vi "Extract subclasses from AUX device.vi"(9 "Data In":string, 10 "Class":string, 11 "Aux Device Settings in":T1 {"Signals"."% Open" min=0.0 max=100.0 step=0.1 format="%.4f"; "Signals"."Position" max=20.0 step=1.0 format="%.4f"; "Speed" max=7 step=1; "Gear" max=7 step=1; "Temp V Err" min=0.0 max=20.0 step=0.1; "Temp Err" min=0.0 max=20.0 step=0.1; "Scaling Factor" min=0.0 max=99.0 step=0.1; "Min Flow" min=0.0 max=20.0 step=0.1}) -> (1 "Data out":string, 3 "Aux Device Settings out":T1 {"Signals"."% Open" min=0.0 max=100.0 step=0.1 format="%.4f"; "Signals"."Position" max=20.0 step=1.0 format="%.4f"; "Speed" max=7 step=1; "Gear" max=7 step=1; "Temp V Err" min=0.0 max=20.0 step=0.1; "Temp Err" min=0.0 max=20.0 step=0.1; "Scaling Factor" min=0.0 max=99.0 step=0.1; "Min Flow" min=0.0 max=20.0 step=0.1})   [LabVIEW 2015, in "Mercury iXX.lvlib" / "Auxiliary.lvlib"]
uses:
  Auxiliary.lvlib
  Controls/AUX Device (Read).ctl
  Controls/Manufacturing Data.ctl
  Controls/AUX Signals (Read).ctl
  Mercury iXX.lvlib
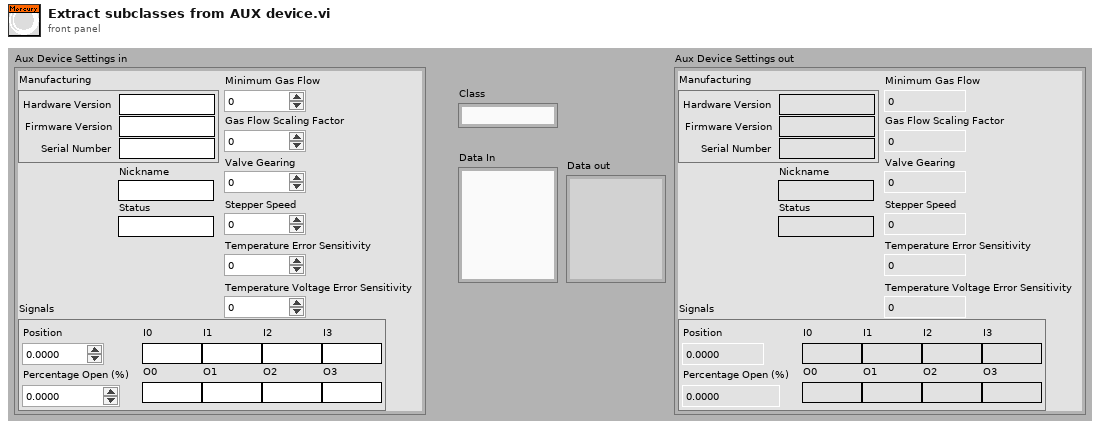
[diagram p1: front panel]
types:
  T1 = typedef "Mercury iXX.lvlib/Auxiliary.lvlib/AUX Device (Read).ctl" = cluster{"Manufacturing":T2, "Min Flow":dbl, "Scaling Factor":dbl, "Temp Err":dbl, "Temp V Err":dbl, "Gear":u32, "Speed":u32, "Signals":T3, "Nickname":string, "Status":string}
  T2 = typedef "Mercury iXX.lvlib/Manufacturing Data.ctl" = cluster{"Hardware Version":string, "Firmware Version":string, "Serial Number":string}
  T3 = typedef "Mercury iXX.lvlib/Auxiliary.lvlib/AUX Signals (Read).ctl" = cluster{"Position":dbl, "% Open":dbl, "I0":string, "I1":string, "I2":string, "I3":string, "O0":string, "O1":string, "O2":string, "O3":string}
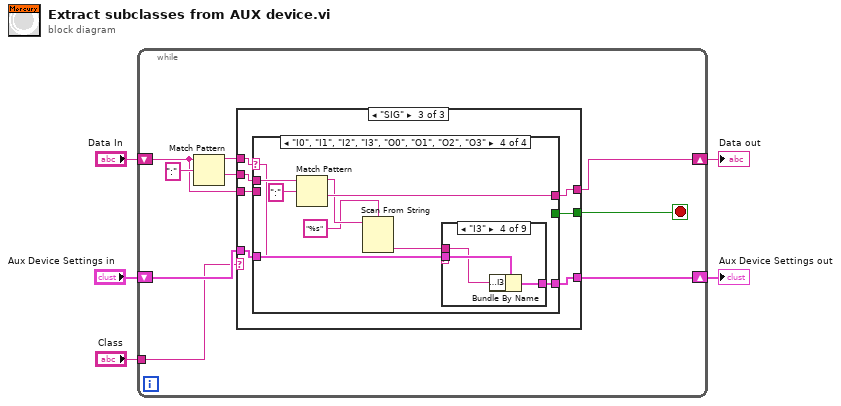
[diagram p0: block diagram]
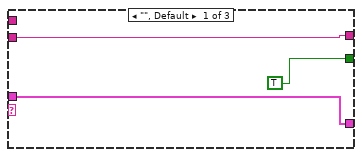
[diagram p2: hidden frame]
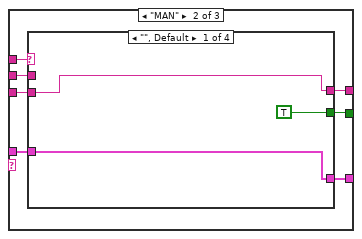
[diagram p3: hidden frame]
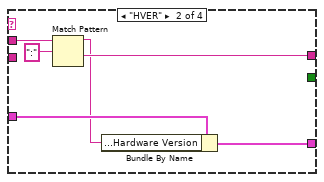
[diagram p4: hidden frame]
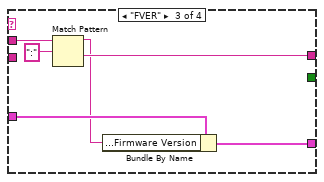
[diagram p5: hidden frame]
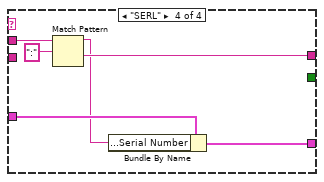
[diagram p6: hidden frame]
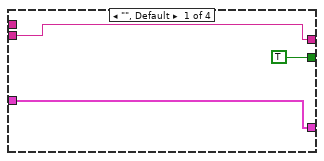
[diagram p7: hidden frame]
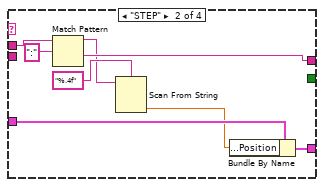
[diagram p8: hidden frame]
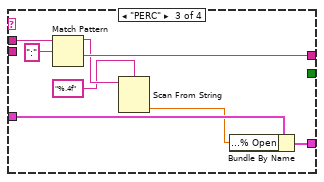
[diagram p9: hidden frame]
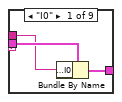
[diagram p10: hidden frame]
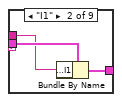
[diagram p11: hidden frame]
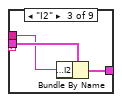
[diagram p12: hidden frame]
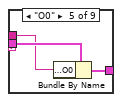
[diagram p13: hidden frame]
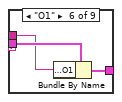
[diagram p14: hidden frame]
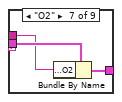
[diagram p15: hidden frame]
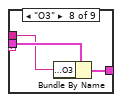
[diagram p16: hidden frame]
diagram:
  n1 = while {
    tunnel: "Class" -> [w8]
    shift-right: [w10] -> w4
    shift-left: "Data In" -> [w6]
    shift-right: [w12] -> w3
    shift-left: "Aux Device Settings in" -> [w13]
    stop <- w7 stop-if-true
    n2 = Match Pattern(string=w6, regular expression=":") -> (before substring=w9:string, after substring=w11:string)  [unwired: 3 out]
    n3 = case shown="\"SIG\"" w8 {
      tunnel: w13 -> [w15 w24 w52]
      tunnel: [w15 w23 w51] -> w12
      tunnel: w11 -> [_ w22 w49]
      tunnel: [w16 w21 w50] -> w10
      tunnel: w9 -> [_ w20 w48]
      tunnel: [TRUE w18 w46] -> w7
      tunnel: w6 -> [w16 w19 w47]
      frame "", Default {
      }
      frame "MAN" {
        n4 = case shown="\"\", Default" w20 {
          tunnel: w24 -> [w27 w33 w39 w45]
          tunnel: [w27 w32 w38 w44] -> w23
          tunnel: w22 -> [_ w31 w37 w43]
          tunnel: [w26 w30 w36 w42] -> w21
          tunnel: w19 -> [w26 _ _ _]
          tunnel: [TRUE _ _ _] -> w18
          frame "", Default {
          }
          frame "HVER" {
            n5 = Match Pattern(string=w31, regular expression=":") -> (before substring=w28:string, after substring=w30:string)  [unwired: 3 out]
            n6 = Bundle By Name(cluster=w33, "Manufacturing.Hardware Version"=w28) -> (w32:T1)
          }
          frame "FVER" {
            n7 = Match Pattern(string=w37, regular expression=":") -> (before substring=w34:string, after substring=w36:string)  [unwired: 3 out]
            n8 = Bundle By Name(cluster=w39, "Manufacturing.Firmware Version"=w34) -> (w38:T1)
          }
          frame "SERL" {
            n9 = Match Pattern(string=w43, regular expression=":") -> (before substring=w40:string, after substring=w42:string)  [unwired: 3 out]
            n10 = Bundle By Name(cluster=w45, "Manufacturing.Serial Number"=w40) -> (w44:T1)
          }
        }
      }
      frame "SIG" {
        n11 = case shown="\"I0\", \"I1\", \"I2\", \"I3\", \"O0\", \"O1\", \"O2\", \"O3\"" w48 {
          selector: w48 -> [_ _ _ w72]
          tunnel: w52 -> [w55 w63 w71 w80]
          tunnel: [w55 w62 w70 w79] -> w51
          tunnel: w49 -> [_ w61 w69 w78]
          tunnel: [w54 w60 w68 w77] -> w50
          tunnel: w47 -> [w54 _ _ _]
          tunnel: [TRUE _ _ _] -> w46
          frame "", Default {
          }
          frame "STEP" {
            n12 = Match Pattern(string=w61, regular expression=":") -> (before substring=w57:string, after substring=w60:string)  [unwired: 3 out]
            n13 = Scan From String(format string="%.4f", input string=w57) -> (output 1=w56:dbl)  [unwired: 2 in, 4 out]
            n14 = Bundle By Name(cluster=w63, "Signals.Position"=w56) -> (w62:T1)
          }
          frame "PERC" {
            n15 = Match Pattern(string=w69, regular expression=":") -> (before substring=w66:string, after substring=w68:string)  [unwired: 3 out]
            n16 = Scan From String(format string="%.4f", input string=w66) -> (output 1=w65:dbl)  [unwired: 2 in, 4 out]
            n17 = Bundle By Name(cluster=w71, "Signals.% Open"=w65) -> (w70:T1)
          }
          frame "I0", "I1", "I2", "I3", "O0", "O1", "O2", "O3" {
            n18 = Match Pattern(string=w78, regular expression=":") -> (before substring=w75:string, after substring=w77:string)  [unwired: 3 out]
            n19 = Scan From String(format string="%s", input string=w75) -> (output 1=w74:string)  [unwired: 2 in, 4 out]
            n20 = case shown="\"I3\"" w72 {
              tunnel: w80 -> [w83 w86 w89 w92 w95 w98 w101 w104 w105]
              tunnel: [w82 w85 w88 w91 w94 w97 w100 w103 w105] -> w79
              tunnel: w74 -> [w81 w84 w87 w90 w93 w96 w99 w102 _]
              frame "I0" {
                n21 = Bundle By Name(cluster=w83, "Signals.I0"=w81) -> (w82:T1)
              }
              frame "I1" {
                n22 = Bundle By Name(cluster=w86, "Signals.I1"=w84) -> (w85:T1)
              }
              frame "I2" {
                n23 = Bundle By Name(cluster=w89, "Signals.I2"=w87) -> (w88:T1)
              }
              frame "I3" {
                n24 = Bundle By Name(cluster=w92, "Signals.I3"=w90) -> (w91:T1)
              }
              frame "O0" {
                n25 = Bundle By Name(cluster=w95, "Signals.O0"=w93) -> (w94:T1)
              }
              frame "O1" {
                n26 = Bundle By Name(cluster=w98, "Signals.O1"=w96) -> (w97:T1)
              }
              frame "O2" {
                n27 = Bundle By Name(cluster=w101, "Signals.O2"=w99) -> (w100:T1)
              }
              frame "O3" {
                n28 = Bundle By Name(cluster=w104, "Signals.O3"=w102) -> (w103:T1)
              }
              frame Default {
              }
            }
          }
        }
      }
    }
  }
  "Data out" <- w4
  "Aux Device Settings out" <- w3
